vi "SNMPSendOID.vi"(0 "IP Address":string="192.168.0.130", 1 "OID":string="1.3.6.1.4.1.318.1.1.12.1.1.0", 5 "Write Community String":string="private", 7 "timeout ms (750)":i32=750, 11 "ErrorIn":errorcluster, 12 "Port Number":u16=161) -> (4 "SNMPDataStrings":string[][](array[string]), 15 "ErrorOut":errorcluster)   [LabVIEW 2012]
panel:
  # ".1.3.6.1.4.1.17095.3.1.0\n.1.3.6.1.4.1.17095.3.2.0"
  # "Int. Temp1 Name\nInt. Temp1 Value"
  # ".1.3.6.1.4.1.17095.3.9.0\n.1.3.6.1.4.1.17095.3.10.0"
  # "Ext. Temp Name\nExt. Temp Value"
  # ".1.3.6.1.4.1.17095.3.13.0\n.1.3.6.1.4.1.17095.3.14.0"
  # "Humidity1 Name\nHumidity1 Value"
  # ".1.3.6.1.4.1.17095.3.17.0\n.1.3.6.1.4.1.17095.3.18.0"
  # "Dew Point Name\nDew Point Value"
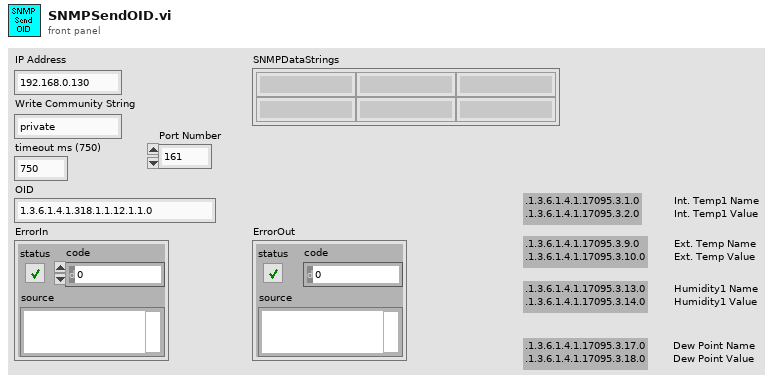
[diagram p1: front panel]
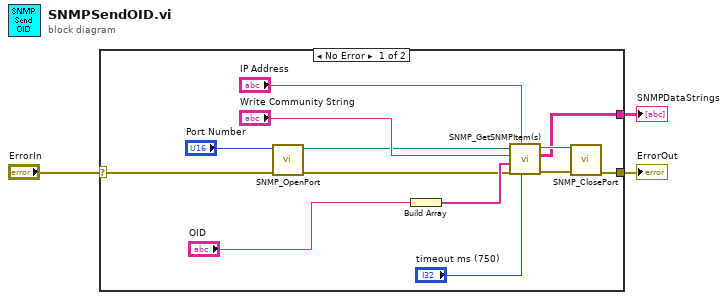
[diagram p0: block diagram]
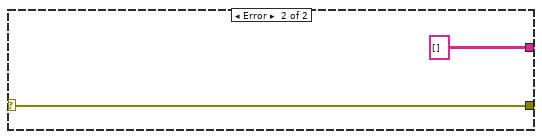
[diagram p2: hidden frame]
diagram:
  n1 = case shown="No Error" "ErrorIn" {
    selector: "ErrorIn" -> [w7 w17]
    tunnel: [w14 w17] -> w3
    tunnel: [w10 string[][] [] ("SnmpDataAsStrings")] -> w2
    frame No Error {
      n2 = call "SNMP_OpenPort.vi"("error in (no error)"=w7, "port"="Port Number") -> ("error out"=w6:errorcluster, "connection ID"=w5:refnum<k16>)  [unwired: 8 out]
      n3 = Build Array("OID") -> (w9:string[])
      n4 = call "SNMP_GetSNMPItem(s).vi"("timeout ms (25000)"="timeout ms (750)", "IP Address of SNMP Device"="IP Address", "error in (no error)"=w6, "OID ARRAY"=w9, "Community Name"="Write Community String", "connection ID in"=w5) -> ("error out"=w15:errorcluster, "SnmpDataAsStrings"=w10:string[][], "connection ID out"=w16:refnum<k16>)  [unwired: 1 in, 2 out]
      n5 = call "SNMP_ClosePort.vi"("error in (no error)"=w15, "connection ID"=w16) -> ("error out"=w14:errorcluster)  [unwired: 9 out]
    }
    frame Error {
    }
  }
  "ErrorOut" <- w3
  "SNMPDataStrings" <- w2
